vi "resample and cut.vi"(5 "new dt":dbl, 7 "signal dt":dbl, 10 "array":dbl[](array[numeric]), 11 "Splite":i32) -> (1 "org second part":waveform(dbl), 2 "resampled first part":waveform(dbl), 3 "Org first part":waveform(dbl))   [LabVIEW 2020]
uses:
  <vilib>/measure/maresamp.llb/Resample Waveform (single shot).vi
  <vilib>/measure/NI_MAPro.lvlib
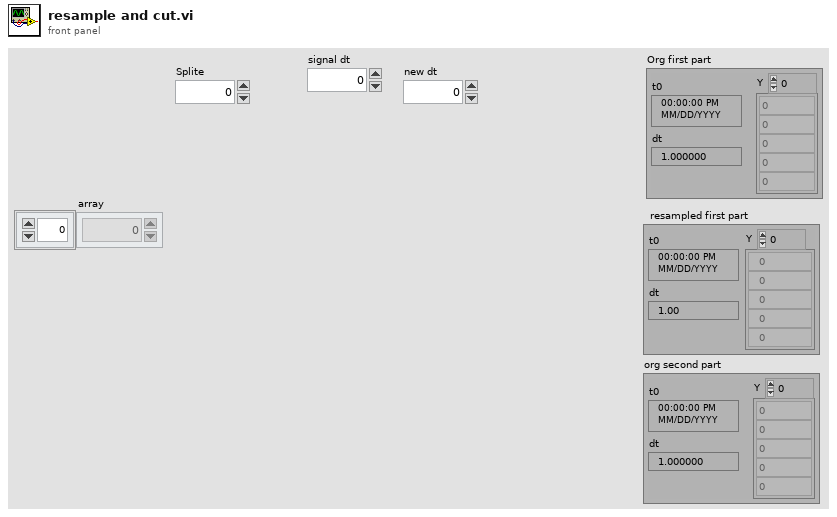
[diagram p1: front panel]
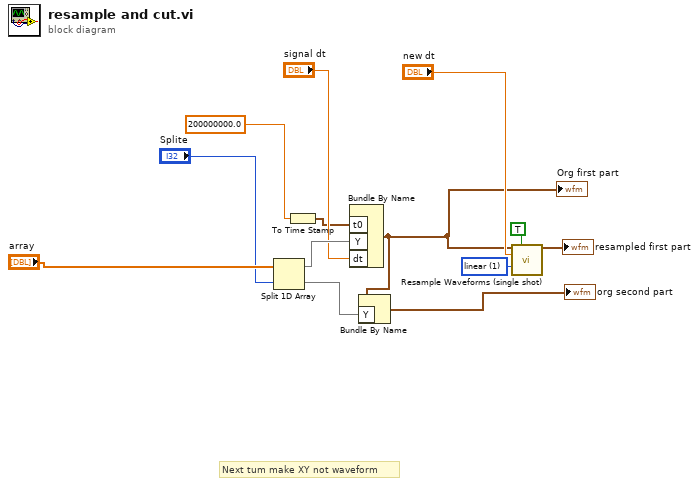
[diagram p0: block diagram]
diagram:
  w10 = u16 1 items=["coerce", "linear", "spline", "FIR filter"] ("interpolation mode")
  # "Next tum make XY not waveform"
  n1 = Split 1D Array(array="array", index="Splite") -> (first subarray=w13:dbl[], second subarray=w12:dbl[])
  n2 = To Time Stamp(1:200000000.0 ("signal dt")) -> (0:w1:timestamp)
  n3 = Bundle By Name("t0"=w1, "Y"=w13, "dt"="signal dt") -> (w3:waveform(dbl))  [unwired: 1 in]
  "Org first part" <- w3
  n4 = Bundle By Name(cluster=w3, "Y"=w12) -> (→"org second part":waveform(dbl))
  n5 = call-poly <vilib>:"Resample Waveforms (single shot).vi"("waveform in"=w3, "open interval? (F)"=TRUE, "dt"="new dt", "interpolation mode"=w10) -> ("resampled waveform out"=→"resampled first part":waveform(dbl))  [unwired: 8 in, 3 out]
